vi "Telnet_Initialize.vi"(8 "error in (no error)":errorcluster, 11 "Address":string="192.168.10.152") -> (0 "error out":errorcluster, 3 "connection ID out":refnum<k5>)   [LabVIEW 2018]
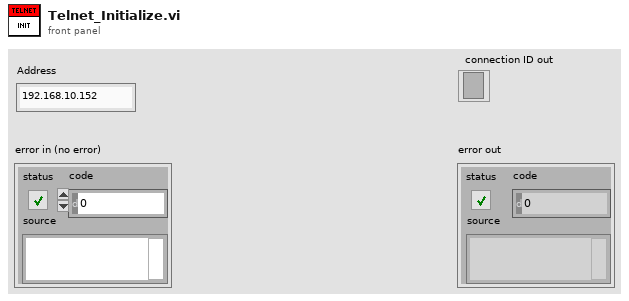
[diagram p1: front panel]
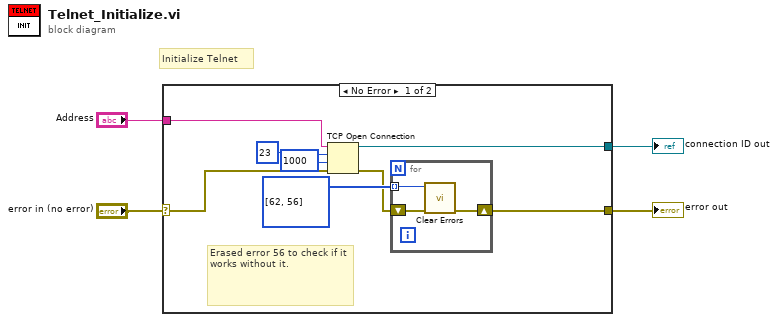
[diagram p0: block diagram]
diagram:
  # "Initialize Telnet"
  n1 = case shown="No Error" "error in (no error)" {
    selector: "error in (no error)" -> [w8 w16]
    tunnel: [w9 _] -> w4
    tunnel: [w7 w16] -> w2
    tunnel: "Address" -> [w6 _]
    frame No Error {
      # "Erased error 56 to check if it works without it."
      n2 = TCP Open Connection(address=w6, remote port or service name=u16 23 ("port"), timeout ms (60000)=1000, error in (no error)=w8) -> (connection ID=w9:refnum<k5>, error out=w5:errorcluster)  [unwired: 1 in]
      n3 = for {
        shift-right: [w14] -> w7
        shift-left: w5 -> [w15]
        tunnel: i32[] [62, 56] -> [w13] mode=indexing
        n4 = call "Clear Errors.vi"("error in (no error)"=w15, "specific error code to clear (0: all)"=w13) -> ("error out"=w14:errorcluster)  [unwired: 4 in, 1 out]
      }
    }
    frame Error {
    }
  }
  "error out" <- w2
  "connection ID out" <- w4
